vi "Create Zip.vi"(4 "Second Zip":path, 6 "ZIP File Name":string, 7 "Generate MD5 File":bool, 8 "error in (no error)":errorcluster, 9 "Top Level VI Path":path, 10 "Destination Directory":path, 11 "Metadata":string) -> (0 "error out":errorcluster, 3 "Zip File Path":path)   [LabVIEW 2014, in "Raspberry Pi Compatible Compiler for LabVIEW.lvlib"]
uses:
  Raspberry Pi Compatible Compiler for LabVIEW.lvlib
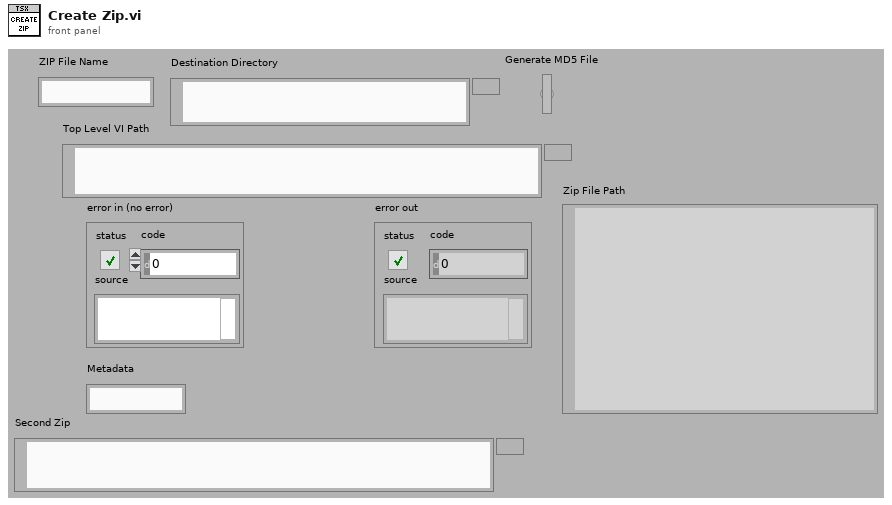
[diagram p1: front panel]
types:
  T1 = enum16{"open", "replace", "create", "open or create", "replace or create", "replace or create with confirmation"}
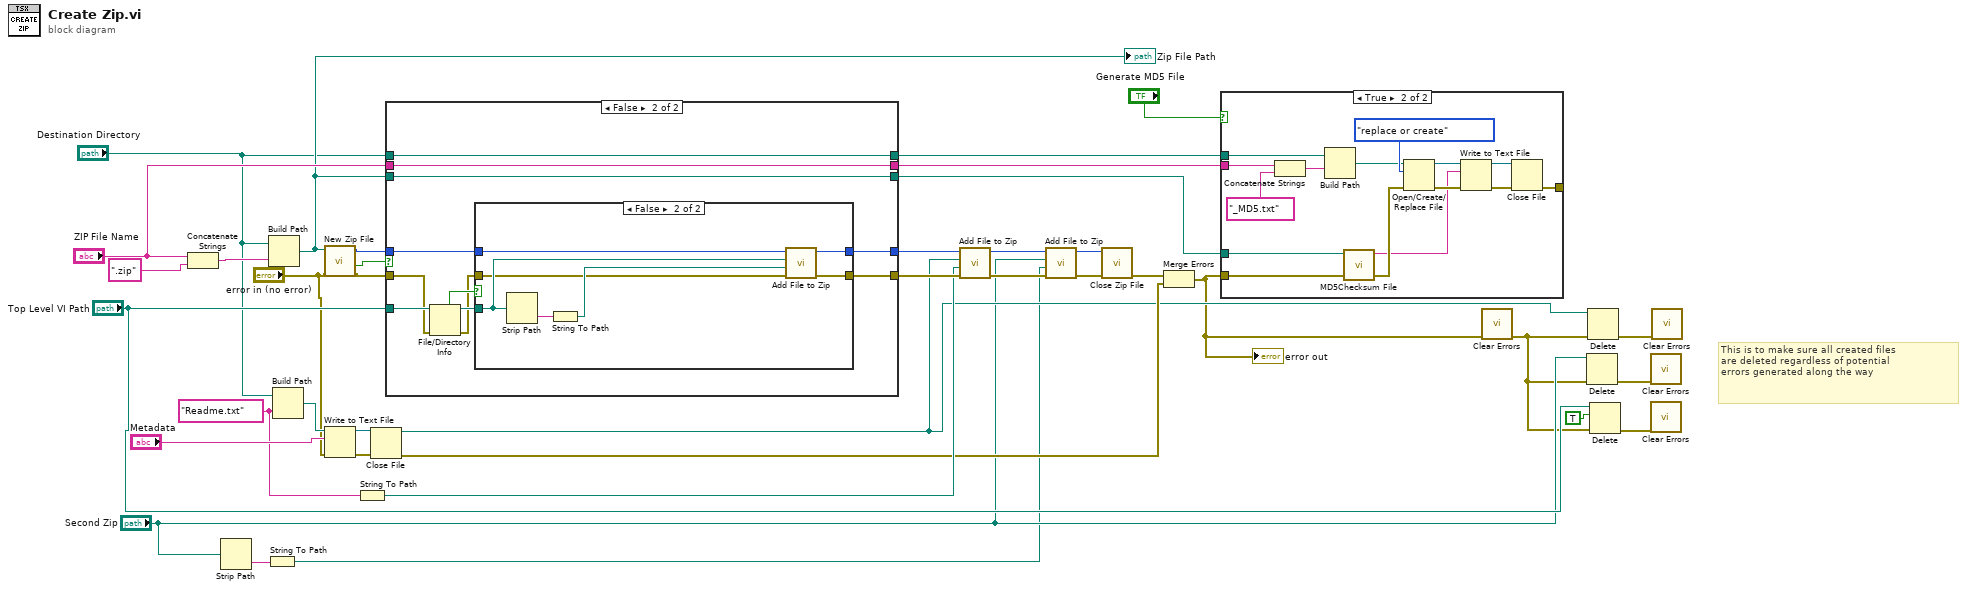
[diagram p0: block diagram]
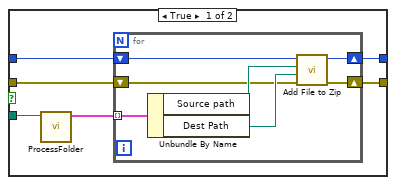
[diagram p4: hidden frame]
diagram:
  w17 = "Readme.txt" ("name or relative path")
  # "This is to make sure all created files\nare deleted regardless of potential\nerrors generated along the way"
  n1 = Concatenate Strings("ZIP File Name", ".zip" ("string")) -> (w32:string)
  n2 = Strip Path(path="Second Zip") -> (name=w8:string)  [unwired: 1 out]
  n3 = String To Path(string=w8) -> (path=w7:path)
  n4 = Build Path(base path="Destination Directory", name or relative path=w32) -> (appended path=w31:path)
  "Zip File Path" <- w31
  n5 = Build Path(base path="Destination Directory", name or relative path=w17) -> (appended path=w24:path)
  n6 = call <vilib>:"New Zip File.vi"("error in (no error)"="error in (no error)", "target"=w31) -> ("error out"=w30:errorcluster, "cancelled"=w29:bool, "zip file out"=w28:i64)  [unwired: 3 in]
  n7 = Write to Text File(file (use dialog)=w24, text="Metadata", error in="error in (no error)") -> (refnum out=w20:refnum<file>, error out=w21:errorcluster)  [unwired: 1 in, 1 out]
  n8 = String To Path(string=w17) -> (path=w16:path)
  n9 = Close File(refnum=w20, error in=w21) -> (path=w10:path, error out=w15:errorcluster)
  n10 = case shown="False" w29 {
    tunnel: w28 -> [w43 w53]
    tunnel: "Top Level VI Path" -> [_ w54]
    tunnel: [w43 w52] -> w19
    tunnel: w30 -> [w42 w45]
    tunnel: [w42 w51] -> w18
    tunnel: w31 -> [w41 w50]
    tunnel: [w41 w50] -> w38
    tunnel: "Destination Directory" -> [w40 w49]
    tunnel: [w40 w49] -> w36
    tunnel: "ZIP File Name" -> [w39 w48]
    tunnel: [w39 w48] -> w35
    frame True {
    }
    frame False {
      n11 = File/Directory Info(path=w54, error in=w45) -> (path out=w47:path, directory=w46:bool, error out=w44:errorcluster)  [unwired: 4 out]
      n12 = case shown="False" w46 {
        tunnel: w53 -> [w58 w74]
        tunnel: [w57 w73] -> w52
        tunnel: w47 -> [w60 w70]
        tunnel: w44 -> [w56 w69]
        tunnel: [w55 w68] -> w51
        frame True {
          n13 = call "ProcessFolder.vi"("Path"=w60) -> ("Array"=w59:cluster{"Source path":path, "Dest Path":path}[])  [unwired: 10 in]
          n14 = for {
            tunnel: w59 -> [w67] mode=indexing
            shift-right: [w61] -> w57
            shift-left: w58 -> [w66]
            shift-right: [w62] -> w55
            shift-left: w56 -> [w63]
            n15 = Unbundle By Name(w67) -> ("Source path"=w65:path, "Dest Path"=w64:path)
            n16 = call <vilib>:"Add File to Zip.vi"("error in (no error)"=w63, "destination path in zip"=w64, "source file path"=w65, "zip file in"=w66) -> ("error out"=w62:errorcluster, "zip file out"=w61:i64)  [unwired: 6 in]
          }
        }
        frame False {
          n17 = Strip Path(path=w70) -> (name=w72:string)  [unwired: 1 out]
          n18 = String To Path(string=w72) -> (path=w71:path)
          n19 = call <vilib>:"Add File to Zip.vi"("error in (no error)"=w69, "destination path in zip"=w71, "source file path"=w70, "zip file in"=w74) -> ("error out"=w68:errorcluster, "zip file out"=w73:i64)  [unwired: 6 in]
        }
      }
    }
  }
  n20 = call <vilib>:"Add File to Zip.vi"("error in (no error)"=w18, "destination path in zip"=w16, "source file path"=w10, "zip file in"=w19) -> ("error out"=w14:errorcluster, "zip file out"=w13:i64)  [unwired: 6 in]
  n21 = call <vilib>:"Add File to Zip.vi"("error in (no error)"=w14, "destination path in zip"=w7, "source file path"="Second Zip", "zip file in"=w13) -> ("error out"=w12:errorcluster, "zip file out"=w11:i64)  [unwired: 6 in]
  n22 = call <vilib>:"Close Zip File.vi"("error in (no error)"=w12, "zip file in"=w11) -> ("error out"=w6:errorcluster)  [unwired: 5 in]
  n23 = Merge Errors(w6, w15) -> (w5:errorcluster)
  "error out" <- w5
  n24 = case shown="True" "Generate MD5 File" {
    tunnel: w38 -> [_ w90]
    tunnel: w5 -> [w75 w89]
    tunnel: w36 -> [_ w80]
    tunnel: [w75 w81] -> _
    tunnel: w35 -> [_ w78]
    frame False {
    }
    frame True {
      n25 = Concatenate Strings(w78, "_MD5.txt" ("name or relative path")) -> (w76:string)
      n26 = Build Path(base path=w80, name or relative path=w76) -> (appended path=w79:path)
      n27 = call <vilib>:"MD5Checksum File.vi"("error in (no error)"=w89, "Path"=w90) -> ("error out"=w88:errorcluster, "MD5 message-digest"=w85:string)  [unwired: 8 in]
      n28 = Open/Create/Replace File(file path (use dialog)=w79, error in=w88, operation (0:open)=T1."replace or create") -> (refnum out=w84:refnum<file>, error out=w86:errorcluster)  [unwired: 3 in, 1 out]
      n29 = Write to Text File(file (use dialog)=w84, text=w85, error in=w86) -> (refnum out=w82:refnum<file>, error out=w83:errorcluster)  [unwired: 1 in, 1 out]
      n30 = Close File(refnum=w82, error in=w83) -> (error out=w81:errorcluster)  [unwired: 1 out]
    }
  }
  n31 = call <vilib>:"Clear Errors.vi"("error in (no error)"=w5) -> ("error out"=w3:errorcluster)  [unwired: 5 in, 1 out]
  n32 = Delete(path (use dialog)="Second Zip", error in=w3) -> (error out=w2:errorcluster)  [unwired: 3 in, 2 out]
  n33 = Delete(path (use dialog)=w10, error in=w3) -> (error out=w4:errorcluster)  [unwired: 3 in, 2 out]
  n34 = Delete(path (use dialog)="Top Level VI Path", entire hierarchy (F)=TRUE, error in=w3) -> (error out=w1:errorcluster)  [unwired: 2 in, 2 out]
  n35 = call <vilib>:"Clear Errors.vi"("error in (no error)"=w2) -> ()  [unwired: 5 in, 2 out]
  n36 = call <vilib>:"Clear Errors.vi"("error in (no error)"=w1) -> ()  [unwired: 5 in, 2 out]
  n37 = call <vilib>:"Clear Errors.vi"("error in (no error)"=w4) -> ()  [unwired: 5 in, 2 out]
